vi "Run Auto Score.vi"(11 "Zip":path) -> (3 "Result":T1)   [LabVIEW 2024, in "Wordle Scorer.lvlib"]
uses:
  Wordle Scorer.lvlib
  Scoring Result.ctl
  Result.ctl
  <vilib>/Utility/error.llb/DialogType.ctl
  b176729e-45e3-4042-bf0b-439ceafae7e1.vi
  10f0845f-5e3d-49fd-8ad4-61868670d3b0.vi
panel:
  out "#":i32
  out "Initial Run Time":dbl format="%_6f"
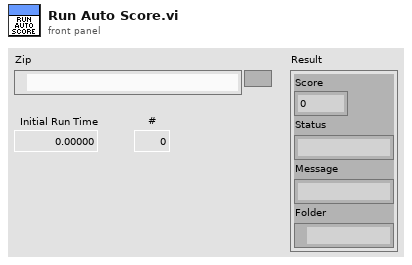
[diagram p1: front panel]
types:
  T1 = typedef "Wordle Scorer.lvlib/Scoring Result.ctl" = cluster{"Score":dbl, "Status":string, "Message":string, "Folder":path}
  T2 = typedef "DialogType.ctl" = u16
  T3 = typedef "Wordle Scorer.lvlib/Result.ctl" = enum16{"failed", "complete", "error", "timeout", "ineligible"}
  T4 = typedef "Word Search Scorer.lvlib/Solver VI Ref Type.ctl" = refnum<vi>
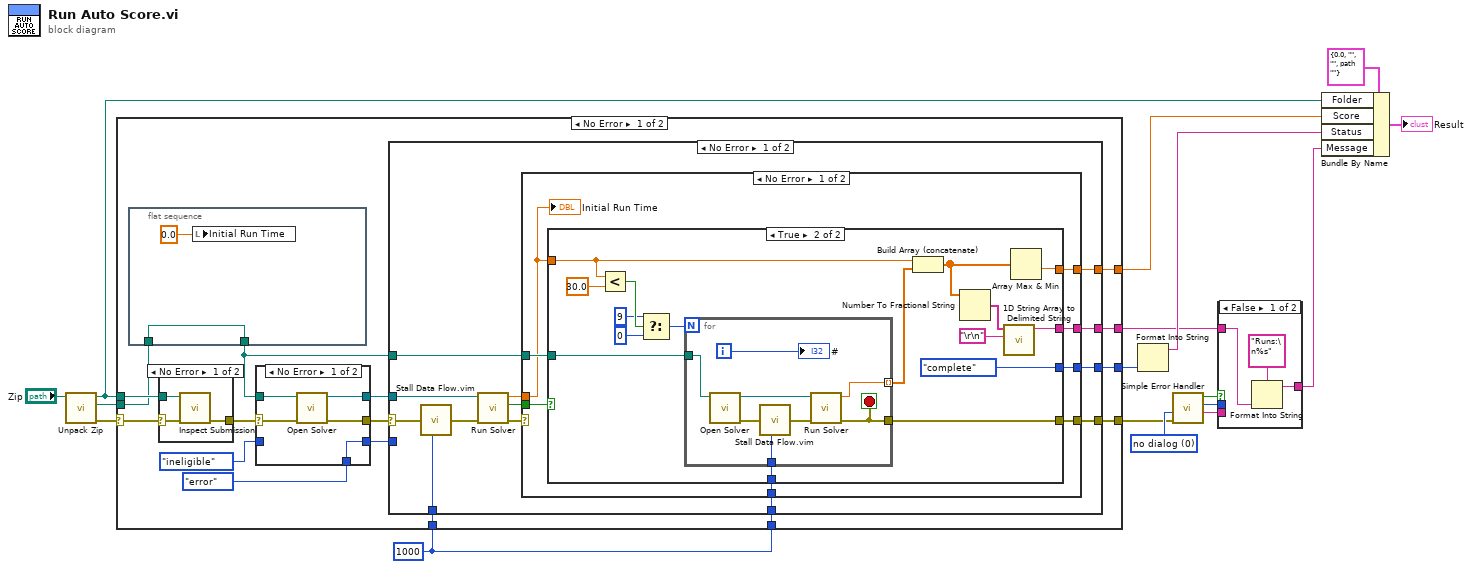
[diagram p0: block diagram]
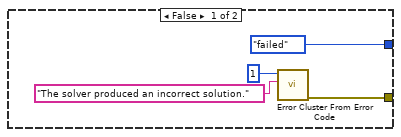
[diagram p2: hidden frame]
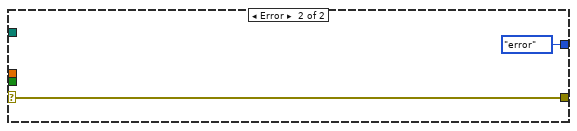
[diagram p3: hidden frame]
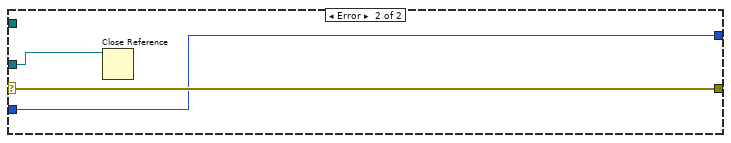
[diagram p4: hidden frame]
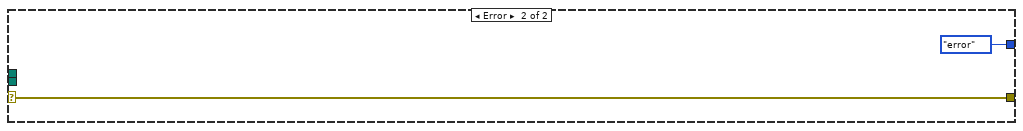
[diagram p7: hidden frame]
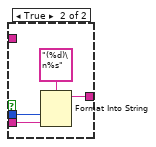
[diagram p8: hidden frame]
diagram:
  w2 = u32 1000 ("milliseconds to wait")
  w9 = T2 0 items=["no dialog", "OK message", "continue or stop message", "OK message + warnings", "continue/stop + warnings"] ("type of dialog (OK msg:1)")
  n1 = call "Unpack Zip.vi"("Zip"="Zip") -> ("error out"=w16:errorcluster, "Solver VI"=w13:path, "Folder"=w5:path)  [unwired: 8 in]
  n2 = case shown="No Error" w16 {
    selector: w16 -> [w33 w101]
    tunnel: w5 -> [w29 _]
    tunnel: w13 -> [w21 _]
    tunnel: [w25 Result."error" ("Result")] -> w8
    tunnel: [w24 w101] -> w7
    tunnel: [w23 _] -> w6
    tunnel: w2 -> [w20 _]
    tunnel: w2 -> [w19 _]
    tunnel: [w18 _] -> w1
    frame No Error {
      n3 = flat-sequence {
        tunnel: [w35] -> w22
        tunnel: w21 -> [w35]
        frame #0 {
          n4 = local write "Initial Run Time"(0.0 ("Initial Run Time")) -> ()
        }
      }
      n5 = case shown="No Error" w33 {
        selector: w33 -> [w98 w100]
        tunnel: w29 -> [w99 _]
        tunnel: [w97 w100] -> w32
        frame No Error {
          n6 = call "Inspect Submission.vi"("error in (no error)"=w98, "Folder"=w99) -> ("error out"=w97:errorcluster)  [unwired: 7 in, 2 out]
        }
        frame Error {
        }
      }
      n7 = case shown="No Error" w32 {
        selector: w32 -> [w93 w96]
        tunnel: w22 -> [w94 _]
        tunnel: [w92 _] -> w30
        tunnel: [w91 w96] -> w31
        tunnel: [w90 w95] -> w27
        tunnel: Result."error" ("Result") -> [w90 _]
        tunnel: Result."ineligible" ("Result") -> [_ w95]
        frame No Error {
          n8 = call "Open Solver.vi"("error in (no error)"=w93, "Solver Path"=w94) -> ("error IO"=w91:errorcluster, "Solver VI"=w92:T4)  [unwired: 8 in]
        }
        frame Error {
        }
      }
      n9 = case shown="No Error" w31 {
        selector: w31 -> [w47 w89]
        tunnel: w30 -> [w48 w88]
        tunnel: [w42 w89] -> w24
        tunnel: w22 -> [w43 _]
        tunnel: [w41 _] -> w23
        tunnel: [w40 w87] -> w25
        tunnel: w27 -> [_ w87]
        tunnel: w20 -> [w38 _]
        tunnel: w19 -> [w37 _]
        tunnel: [w36 _] -> w18
        frame No Error {
          n10 = call "Stall Data Flow.vim"("value in"=w47, "milliseconds to wait"=w38) -> ("value out"=w39:errorcluster)  [unwired: 1 out]
          n11 = call "Run Solver.vi"("error in (no error)"=w39, "Solver VI"=w48) -> ("error out"=w46:errorcluster, "Completed"=w45:bool, "Run Time"=w44:dbl)  [unwired: 7 in]
          n12 = case shown="No Error" w46 {
            selector: w46 -> [_ w86]
            tunnel: w45 -> [w56 _]
            tunnel: w44 -> [w51 _]
            tunnel: w43 -> [w55 _]
            tunnel: [w54 w86] -> w42
            tunnel: [w53 _] -> w41
            tunnel: [w52 Result."error" ("Result")] -> w40
            tunnel: w37 -> [w50 _]
            tunnel: [w49 _] -> w36
            frame No Error {
              n13 = case shown="True" w56 {
                tunnel: w51 -> [_ w70]
                tunnel: w55 -> [_ w72]
                tunnel: [w59 w71] -> w54
                tunnel: [_ w65] -> w53
                tunnel: [Result."failed" ("Result") Result."complete" ("Result")] -> w52
                tunnel: w50 -> [_ w67]
                tunnel: [_ w62] -> w49
                frame False {
                  n14 = call <vilib>:"Error Cluster From Error Code.vi"("error message (\"\")"="The solver produced an incorrect solution.", "error code (0)"=1) -> ("error out"=w59:errorcluster)  [unwired: 7 in]
                }
                frame True {
                  n15 = Less?(x=w70, y=30.0) -> (x < y?=w75:bool)
                  n16 = Select(t=9, s=w75, f=0) -> (s? t:f=w66:i32)
                  n17 = for {
                    N: w66 -> [_]
                    tunnel: w72 -> [w82]
                    tunnel: [w81] -> w71
                    tunnel: [w80] -> w69 mode=indexing
                    tunnel: w67 -> [w77]
                    i -> [w79]
                    stop <- w81 stop-if-true
                    n18 = call "Open Solver.vi"("Solver Path"=w82) -> ("error IO"=w83:errorcluster, "Solver VI"=w84:T4)  [unwired: 9 in]
                    n19 = call "Stall Data Flow.vim"("value in"=w83, "milliseconds to wait"=w77) -> ("value out"=w78:errorcluster)  [unwired: 1 out]
                    n20 = call "Run Solver.vi"("error in (no error)"=w78, "Solver VI"=w84) -> ("error out"=w81:errorcluster, "Run Time"=w80:dbl)  [unwired: 7 in, 1 out]
                    "#" <- w79
                  }
                  n21 = Build Array (concatenate)(w70, w69) -> (w64:dbl[])
                  n22 = Number To Fractional String(number=w64) -> (F-format string=w63:string[])  [unwired: 3 in]
                  n23 = call <vilib>:"1D String Array to Delimited String.vi"("delimiter"="\r\n", "string array"=w63) -> ("delimited string"=w62:string)  [unwired: 9 in]
                  n24 = Array Max & Min(array=w64) -> (min value=w65:dbl)  [unwired: 3 out]
                }
              }
              "Initial Run Time" <- w51
            }
            frame Error {
            }
          }
        }
        frame Error {
          n25 = Close Reference(reference=w88) -> ()  [unwired: 1 in, 1 out]
        }
      }
    }
    frame Error {
    }
  }
  n26 = Format Into String(w8) -> (resulting string=w4:string)  [unwired: 3 in, 1 out]
  n27 = call <vilib>:"Simple Error Handler.vi"("type of dialog (OK msg:1)"=w9, "error in (no error)"=w7) -> ("error?"=w12:bool, "code out"=w11:i32, "source out"=w10:string)  [unwired: 3 in, 2 out]
  n28 = case shown="False" w12 {
    tunnel: w10 -> [_ w107]
    tunnel: w11 -> [_ w108]
    tunnel: w1 -> [w105 _]
    tunnel: [w103 w106] -> w3
    frame False {
      n29 = Format Into String(format string="Runs:\n%s", w105) -> (resulting string=w103:string)  [unwired: 2 in, 1 out]
    }
    frame True {
      n30 = Format Into String(format string="(%d)\n%s", w108, w107) -> (resulting string=w106:string)  [unwired: 2 in, 1 out]
    }
  }
  n31 = Bundle By Name(cluster=T1 {"Score"=0.0, "Status"="", "Message"="", "Folder"=path ""} ("Scoring Result"), "Folder"=w5, "Score"=w6, "Status"=w4, "Message"=w3) -> (→"Result":T1)
